vi "Actor Core.vi"(8 "error in":errorcluster, 11 "CS++GoBangServer in":refnum<class "CS++GoBangServer.lvclass">) -> (0 "error out":errorcluster, 3 "Actor out":refnum<class "Actor.lvclass">)   [LabVIEW 2013, in "GoBang.lvlib" / "CS++GoBangServer.lvclass"]
doc: "(<B>Filename</B>: Actor Framework.lvlib:Actor.lvclass:Actor Core.vi)\n\nReceives messages to the actor, reacts to them, and initiates any error handling that may shut the actor down.\n\nDescendant classes may override this VI to append parallel tasks for the actor to complete while it handles messages. Overrides use the Call Parent Method node."
uses:
  CS++GoBangServer.lvclass
  <vilib>/ActorFramework/Actor/Actor.lvclass
  Core/Actors/CS++SVMonitor/CS++SVMonitor.lvclass
  CS++GoBangServer Messages/JoinGame Msg/JoinGame Msg.lvclass
  CS++GoBangServer Messages/Analyse Board Msg/Analyse Board Msg.lvclass
  Core/Classes/CS++ProcessVariables/SVConnection/SVConnection.lvclass
  Core/Classes/CS++ProcessVariables/PVConnection/PVConnection.lvclass
  CS++GoBangServer.lvclass/CS++GoBangServer.ctl
  Core/Classes/CS++ProcessVariables/PVConnection/PVConnection.lvclass/PVConnection.ctl
  Core/Actors/CS++BaseActor/CS++BaseActor.lvclass/CS++BaseActor.ctl
  <vilib>/ActorFramework/Actor/Actor.lvclass/Actor.ctl
  <vilib>/ActorFramework/Message Enqueuer/Message Enqueuer.lvclass/Message Enqueuer.ctl
  Core/Actors/CS++PVMonitor/CS++PVMonitor.lvclass/CS++PVMonitor.ctl
  Core/Actors/CS++PVMonitor Messages/Register PVs Msg/Register PVs Msg.lvclass/Register PVs Msg.ctl
  Core/Actors/CS++BaseActor/CS++BaseActor.lvclass
  <vilib>/ActorFramework/Message Enqueuer/Init from Existing Queue.vi
  <vilib>/ActorFramework/Message Enqueuer/Enqueue.vi
  <vilib>/ActorFramework/Message Priority Queue/Priority Enqueue.vi
  <vilib>/ActorFramework/Message Enqueuer/Message Enqueuer.lvclass
  Core/Actors/CS++PVMonitor Messages/Register PVs Msg/Register PVs Msg.lvclass
  Core/Actors/CS++PVMonitor/CS++PVMonitor.lvclass
  GoBang.lvlib
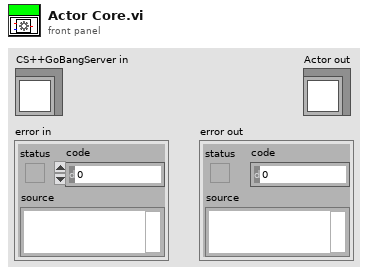
[diagram p1: front panel]
types:
  T1 = enum32{"Invalid", "Standard", "Closed", "Hidden", "Minimized", "Maximized"}
  T2 = cluster{"UpdateBoard":string, "\nAnalyse Board Msg.lvclass":refnum<class "Analyse Board Msg.lvclass">}
  T3 = cluster{"JoinGame":string, "JoinGame Msg.lvclass":refnum<class "JoinGame Msg.lvclass">}
  T4 = cluster{"UpdateBoard":string, "\nAnalyse Board Msg.lvclass":refnum<class "CS++PVUpdate Msg.lvclass">}[]
  T5 = cluster{"Self Enqueuer":refnum<class "Message Enqueuer.lvclass">, cluster{"UpdateBoard":string, "\nAnalyse Board Msg.lvclass":refnum<class "CS++PVUpdate Msg.lvclass">}[]}
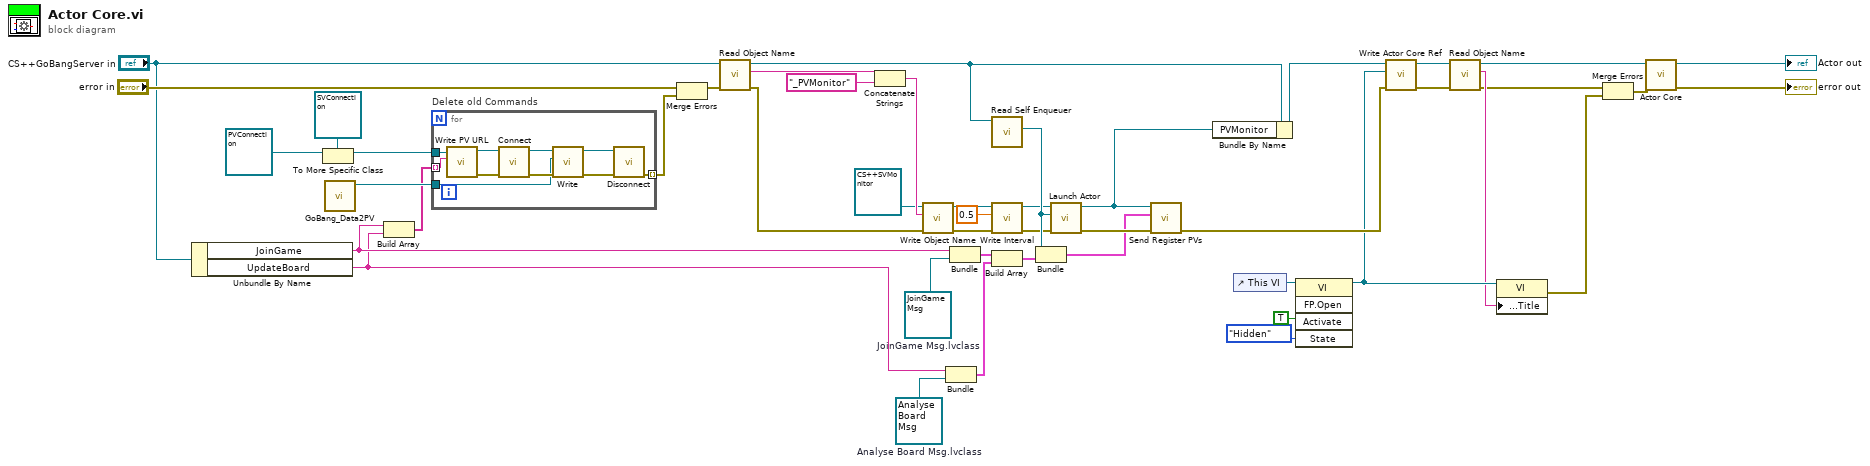
[diagram p0: block diagram]
diagram:
  w28 = refnum<class "Analyse Board Msg.lvclass"> refnum  # Analyse Board Msg.lvclass
  w29 = refnum<class "JoinGame Msg.lvclass"> refnum  # JoinGame Msg.lvclass
  n1 = Unbundle By Name("CS++GoBangServer in") -> ("JoinGame"=w3:string, "UpdateBoard"=w2:string)
  n2 = To More Specific Class(target class=refnum<class "SVConnection.lvclass"> refnum ("CS++ProcessVariables.lvlib:SVConnection.lvclass"), reference=refnum<class "PVConnection.lvclass"> refnum ("CS++ProcessVariables.lvlib:PVConnection.lvclass")) -> (specific class reference=w7:refnum<class "SVConnection.lvclass">)  [unwired: 1 in, 1 out]
  n3 = call "GoBang_Data2PV.vi"() -> ("PV out"=w6:refnum<class "PV.lvclass">)  [unwired: 11 in]
  n4 = Build Array(w3, w2) -> (w1:string[])
  n5 = for "Delete old Commands" {
    tunnel: w7 -> [w56]
    tunnel: w6 -> [w49]
    tunnel: [w48] -> w4 mode=indexing
    tunnel: w1 -> [w47] mode=indexing
    n6 = call "Write PV URL.vi"("PV URL"=w47, "PVConnection in"=w56) -> ("error out"=w52:errorcluster, "PVConnection out"=w55:refnum<class "SVConnection.lvclass">)  [unwired: 8 in]
    n7 = call-dynamic "Connect.vi"("error in (no error)"=w52, "PVConnection in"=w55) -> ("error out"=w51:errorcluster, "PVConnection out"=w54:refnum<class "SVConnection.lvclass">)  [unwired: 8 in]
    n8 = call-dynamic "Write.vi"("error in (no error)"=w51, "PV"=w49, "PVConnection in"=w54) -> ("error out"=w50:errorcluster, "PVConnection out"=w53:refnum<class "SVConnection.lvclass">)  [unwired: 7 in]
    n9 = call-dynamic "Disconnect.vi"("error in (no error)"=w50, "PVConnection in"=w53) -> ("error out"=w48:errorcluster)  [unwired: 8 in, 1 out]
  }
  n10 = Merge Errors("error in", w4) -> (w5:errorcluster)
  n11 = call "Read Object Name.vi"("error in (no error)"=w5, "CS++BaseActor in"="CS++GoBangServer in") -> ("error out"=w25:errorcluster, "Object Name"=w33:string, "CS++BaseActor out"=w32:refnum<class "CS++GoBangServer.lvclass">)  [unwired: 7 in]
  n12 = Concatenate Strings(w33, "_PVMonitor" ("Object Name")) -> (w38:string)
  n13 = call "Write Object Name.vi"("error in (no error)"=w25, "Object Name"=w38, "CS++BaseActor in"=refnum<class "CS++SVMonitor.lvclass"> refnum ("CS++SVMonitor.lvlib:CS++SVMonitor.lvclass")) -> ("error out"=w35:errorcluster, "CS++BaseActor out"=w37:refnum<class "CS++SVMonitor.lvclass">)  [unwired: 7 in]
  n14 = Bundle("UpdateBoard"=w2, "Analyse Board Msg.lvclass"=w28) -> (w27:T2)  [unwired: 1 in]
  n15 = Bundle("JoinGame"=w3, "JoinGame Msg.lvclass"=w29) -> (w44:T3)  [unwired: 1 in]
  n16 = call <vilib>:"Read Self Enqueuer.vi"("Actor"=w32) -> ("Self Enqueuer"=w42:refnum<class "Message Enqueuer.lvclass">)  [unwired: 10 in]
  n17 = call "Write Interval.vi"("error in (no error)"=w35, "Interval"=dbl[unit] 0.5, "CS++PVMonitor in"=w37) -> ("error out"=w24:errorcluster, "CS++PVMonitor out"=w39:refnum<class "CS++SVMonitor.lvclass">)  [unwired: 7 in]
  n18 = Build Array(w44, w27) -> (w43:T4)
  n19 = Bundle("Self Enqueuer"=w42, w43) -> (w30:T5)  [unwired: 1 in]
  n20 = call <vilib>:"Launch Actor.vi"("error in (no error)"=w24, "Actor-to-Caller Enqueuer"=w42, "Actor"=w39) -> ("error out"=w31:errorcluster, "Caller-To-Actor Enqueuer"=w26:refnum<class "Message Enqueuer.lvclass">)  [unwired: 7 in]
  n21 = call "Send Register PVs.vi"("error in (no error)"=w31, "Register Info"=w30, "Message Enqueuer"=w26) -> ("error out"=w22:errorcluster)  [unwired: 7 in, 1 out]
  n22 = Bundle By Name(cluster=w32, "PVMonitor"=w26) -> (w23:refnum<class "CS++GoBangServer.lvclass">)
  n23 = control-ref of="This VI"() -> (w19:refnum<vi>)
  n24 = invoke class="VI" method="FP.Open"(reference=w19, "Activate"=TRUE ("Activate?"), "State"=T1."Hidden") -> (reference out=w16:refnum<vi>)  [unwired: 2 in, 4 out]
  n25 = call "Write Actor Core Ref.vi"("error in (no error)"=w22, "Actor Core Ref"=w16, "CS++BaseActor in"=w23) -> ("error out"=w17:errorcluster, "CS++BaseActor out"=w18:refnum<class "CS++GoBangServer.lvclass">)  [unwired: 7 in]
  n26 = call "Read Object Name.vi"("error in (no error)"=w17, "CS++BaseActor in"=w18) -> ("error out"=w12:errorcluster, "Object Name"=w15:string, "CS++BaseActor out"=w13:refnum<class "CS++GoBangServer.lvclass">)  [unwired: 7 in]
  n27 = property class="VI"(reference=w16, "Front Panel.Title"=w15) -> (error out=w14:errorcluster)  [unwired: 1 in, 1 out]
  n28 = Merge Errors(w12, w14) -> (w11:errorcluster)
  n29 = call-parent "Actor Core.vi"("error in"=w11, "CS++BaseActor in"=w13) -> ("error out"=→"error out":errorcluster, "Actor out"=→"Actor out":refnum<class "Actor.lvclass">)  [unwired: 8 in]
